vi "Prédiction température.vi"(8 "Temps -2":dbl, 9 "Temps -1":dbl, 11 "Temps 0":dbl) -> (1 "Temps-1":dbl format="%#_13g", 3 "Temps pred":dbl)   [LabVIEW 2018]
uses:
  <vilib>/imath/engines/lvmath2/RunTimeEngine/Managers/WorkSpace/UID Generator.vi
  <vilib>/imath/engines/lvmath2/RunTimeEngine/RunTimeType/NIMS_RunTimeType_From StrictType (excl LVString).vi
  <instcachedir>/0/NIMS_RunTimeType_From StrictType (excl LVString)_E7E34A65C99947108168652BAD14964D.lvgen/NIMS_RunTimeType_From StrictType (excl LVString)_E7E34A65C99947108168652BAD14964D_000.vi
  <vilib>/imath/engines/lvmath2/RunTimeEngine/LocalVariableDefStatement/MC_LocalVariableDefStatement_Display.vi
  <vilib>/imath/engines/lvmath2/RunTimeEngine/Managers/SymbolTable/Clear UID.vi
  <vilib>/imath/engines/lvmath2/RunTimeEngine/NodeEndStatement/NIMS_NodeEndStatement_Output.vi
  <instcachedir>/0/NIMS_NodeEndStatement_Output_53EC0D466D134D7ABD903AC30B43404B.lvgen/NIMS_NodeEndStatement_Output_53EC0D466D134D7ABD903AC30B43404B_009.vi
  <vilib>/imath/engines/lvmath2/RunTimeEngine/ErrorHandling/NIMS_Finalize Error.vi
  <vilib>/imath/engines/lvmath2/RunTimeEngine/Managers/SymbolTable/NIMS_WorkSpace.lvlib
panel:
  out "tau":dbl
  # "devient la prédite"
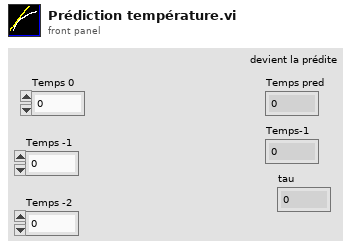
[diagram p1: front panel]
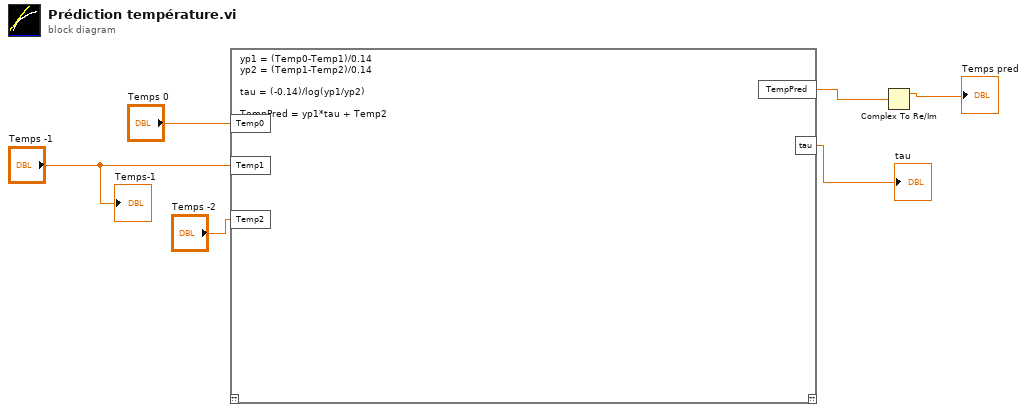
[diagram p0: block diagram]
diagram:
  n1 = mathscript code="yp1 = (Temp0-Temp1)/0.14\nyp2 = (Temp1-Temp2)/0.14\n\ntau = (-0.14)/log(yp1/yp2)\n\nTempPred = yp1*tau + Temp2"("Temp0"="Temps 0", "Temp1"="Temps -1", "Temp2"="Temps -2") -> ("TempPred"=w3:cdb, "tau"=→"tau":cdb)  [unwired: 1 in, 1 out]
  n2 = Complex To Re/Im(x + iy=w3) -> (x=→"Temps pred":dbl)  [unwired: 1 out]
  "Temps-1" <- "Temps -1"
